vi "Method_Const.vi"(4 "Value":dbl, 5 "Value A":refnum<class "Abs_Double Float.lvclass">) -> (1 "Result":refnum<class "Abs_Boolean.lvclass">)   [LabVIEW 2021, in "Equal_DBL.lvclass"]
uses:
  Equal_DBL.lvclass
  Abs_Types/Double Float/Abs_Double Float.lvclass
  Abs_Types/Boolean/Abs_Boolean.lvclass
  C:/TSA/LV_Abstract/Source/Functions/Support/Compare/Two Term/DBL/AbsComp_Two Term_DBL.lvclass
  C:/Program Files (x86)/National Instruments/LabVIEW 2021/vi.lib/TSA/Abstract Data Classes/Abs_Types/Boolean/Abs_Boolean.lvclass
  Support/Compare/Two Term/DBL/AbsComp_Two Term_DBL.lvclass/AbsComp_Two Term_DBL.ctl
  Support/Compare/Two Term/DBL/Properties/Write Numeric A.vi
  Support/Compare/Two Term/DBL/Properties/Write Numeric B.vi
  Constants/Support/DBL/Const_DBL.lvclass
  C:/Program Files (x86)/National Instruments/LabVIEW 2021/vi.lib/TSA/Abstract Data Classes/Abs_Types/Numeric/Abs_Numeric.lvclass
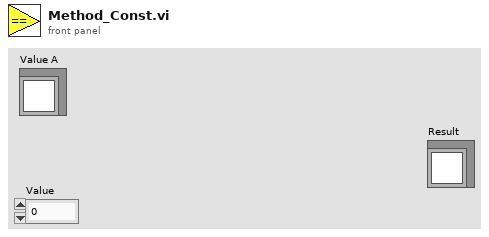
[diagram p1: front panel]
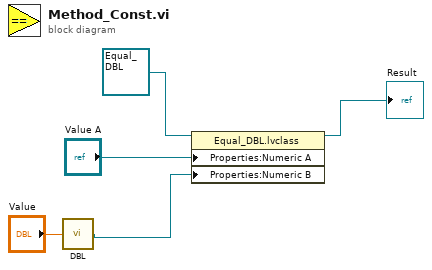
[diagram p0: block diagram]
diagram:
  n1 = call "DBL.vi"("Value"="Value") -> ("Constant"=w2:refnum<class "Const_DBL.lvclass">)  [unwired: 4 in]
  n2 = property class="Equal_DBL.lvclass"(reference=refnum<class "Equal_DBL.lvclass"> refnum ("Greater 0_U64.lvclass"), "Properties:Numeric A"="Value A", "Properties:Numeric B"=w2) -> (reference out=→"Result":refnum<class "Equal_DBL.lvclass">)  [unwired: 1 in, 1 out]
